vi "07_dosing.vi"() -> ()   [LabVIEW 2024]
uses:
  <vilib>/Utility/error.llb/DialogType.ctl
  4067e6f5-c9bb-441e-8d38-abed3cce061a.vi
  <vilib>/Waveform/WDTOps.llb/WDT Get XY Value DBL.vi
  <vilib>/Utility/file.llb/Write Delimited Spreadsheet (DBL).vi
  <instrlib>/Tektronix DMM40x0 Series/Tektronix DMM40x0 Series.lvlib
panel:
  in  "stop":bool
  out "STABLE":bool
  in  "Serial Communication":T1={"Baud Rate"=9600, "Parity"=0, "Data Bits"=8, "Stop Bits"=10, "Flow Control"=0} {"Flow Control" items=["None", "XON/XOFF", "RTS/CTS", "XON/XOFF & RTS/CTS", "DTR/DSR", "XON/XOFF & DTR/DSR"]; "Stop Bits" items=["1.0"=10, "1.5"=15, "2.0"=20]; "Data Bits" items=["7"=7, "8"=8]; "Parity" items=["None", "Odd", "Even", "Mark", "Space"]; "Baud Rate" items=["300"=300, "600"=600, "1200"=1200, "2400"=2400, "4800"=4800, "9600"=9600, "19200"=19200]}
  out "Stability threshold":dbl format="%#_13g"
  out "Waveform Graph":dbl[](graph)
  # "Voltmeter Serial Configuration"
  # "DEFAULT SETTINGS:\n\nTimeout (10000 ms)\nTrigger Count (5000)\nSample Count (1)\n\n****DC VOLTAGE***"
  # "Voltmeter Stability"
  # "0 - Stability threshold not met\n1 - Stability threshold met\n\n\n\n*stability (+/-0.05 mV) of last 15 pts"
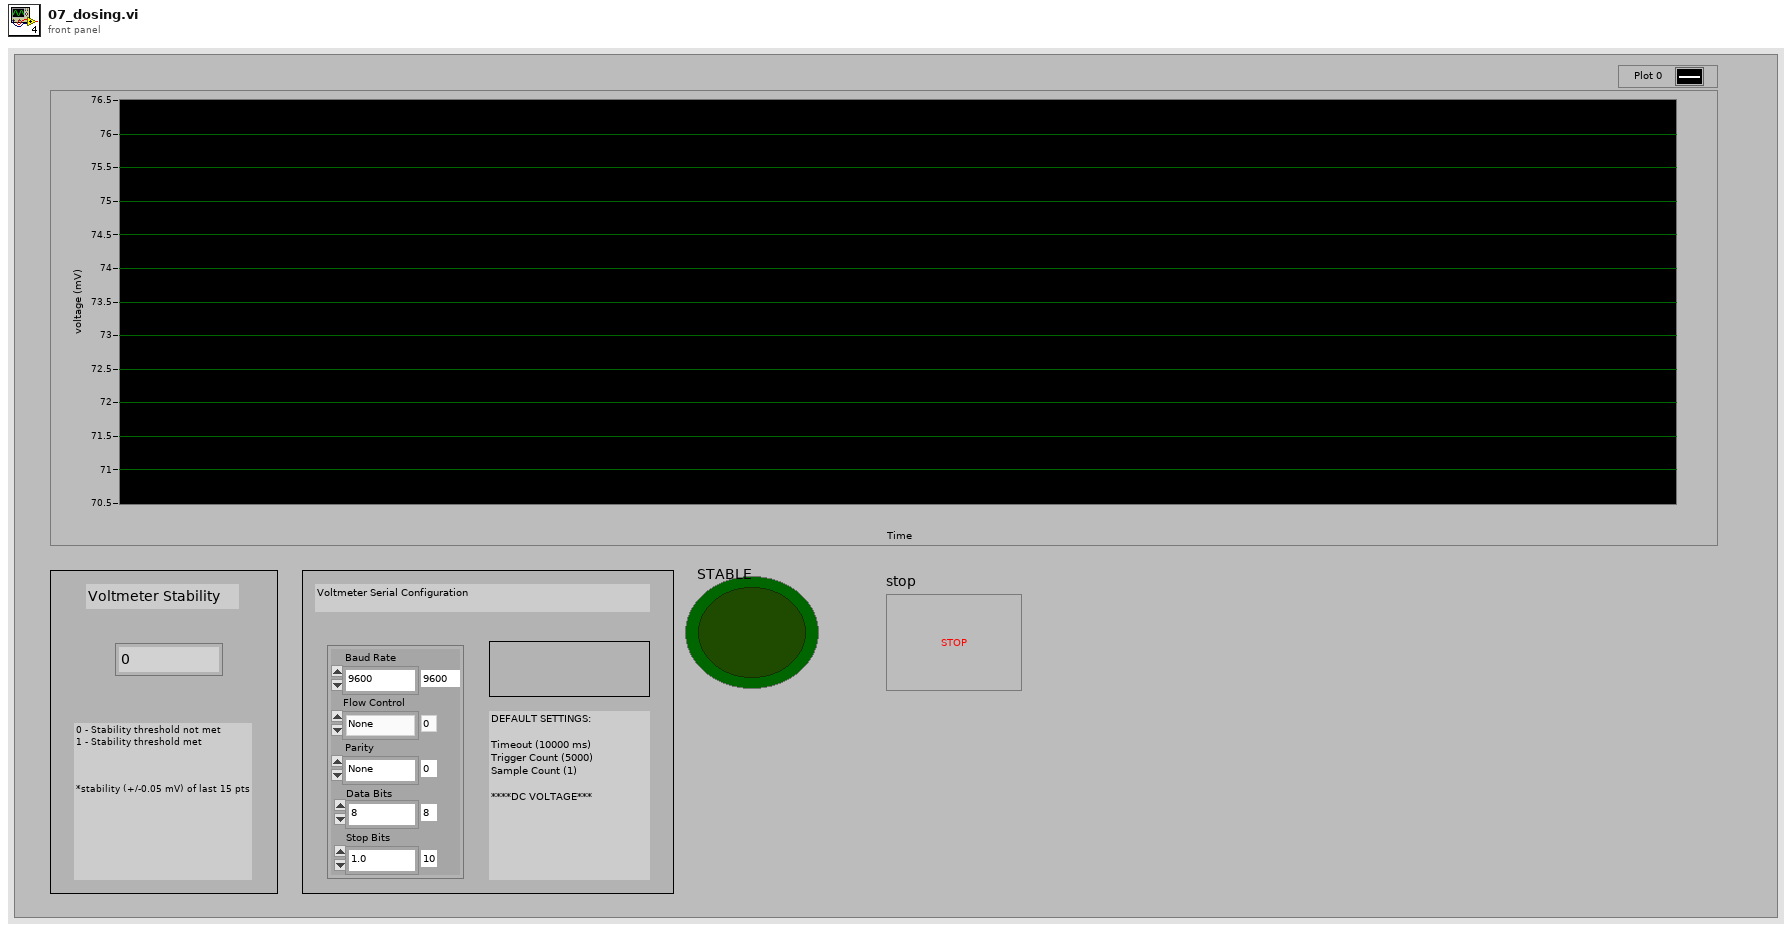
[diagram p1: front panel]
types:
  T1 = cluster{"Baud Rate":u32, "Parity":u16, "Data Bits":u16, "Stop Bits":u16, "Flow Control":u16}
  T2 = typedef "DialogType.ctl" = u16
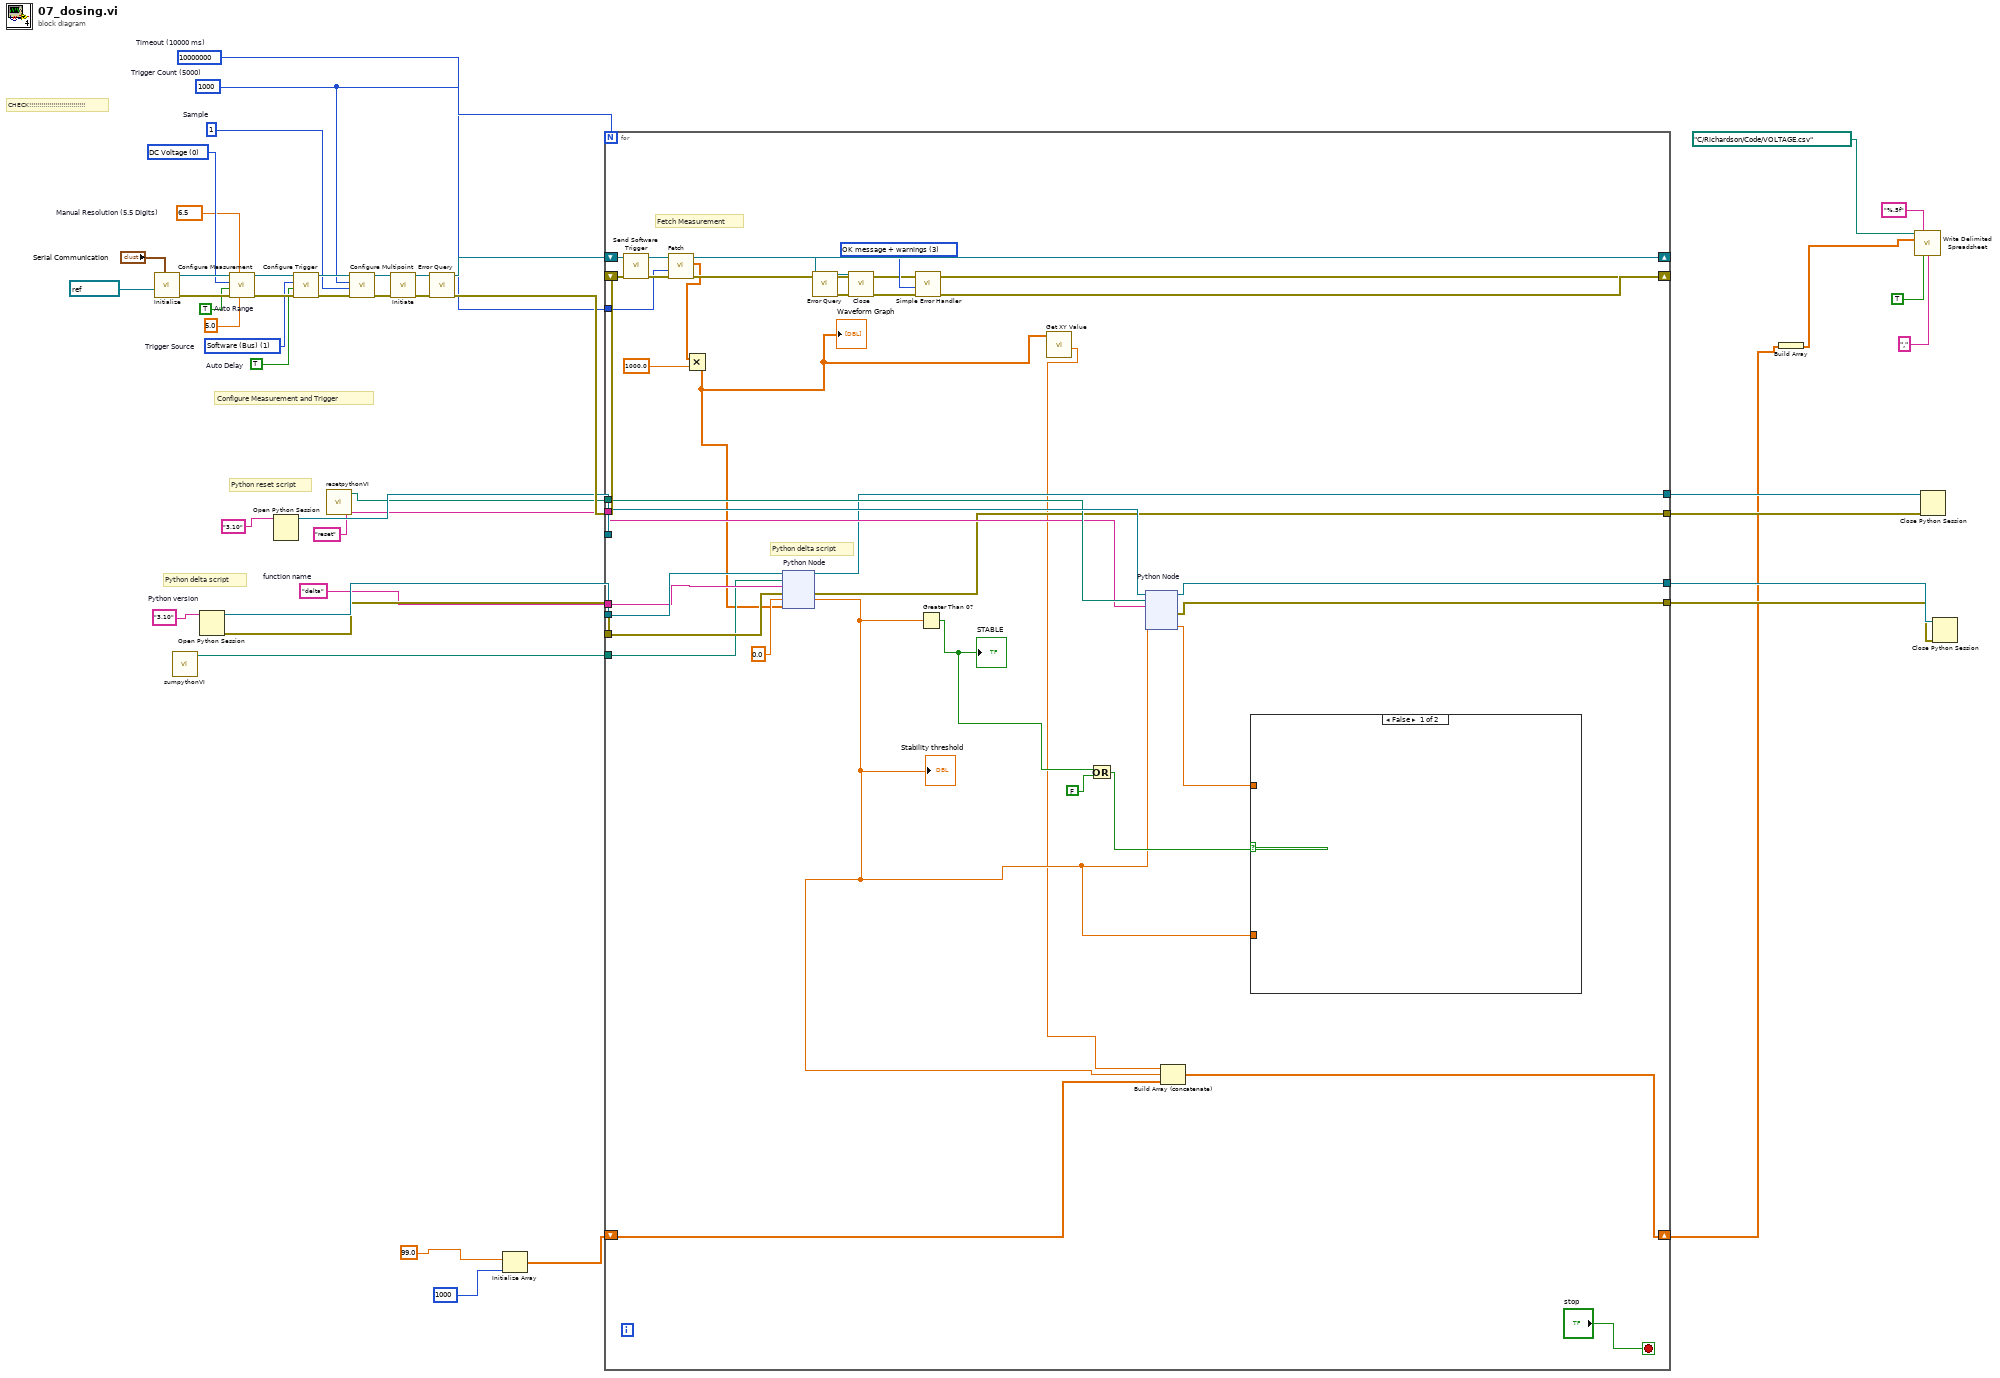
[diagram p0: block diagram]
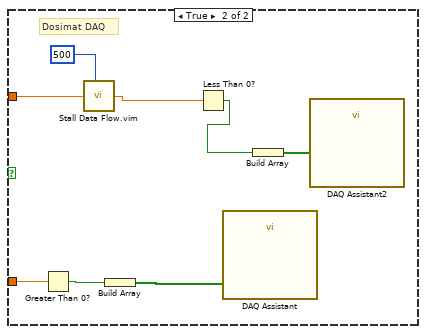
[diagram p2: hidden frame]
diagram:
  w10 = T2 3 items=["no dialog", "OK message", "continue or stop message", "OK message + warnings", "continue/stop + warnings"] ("type of dialog (OK msg:1)")
  w23 = "delta"  # function name
  w26 = "3.10"  # Python version
  w38 = u16 0 items=["DC Voltage", "AC Voltage", "2 - Wire Resistance", "4 - Wire Resistance", "DC Current", "AC Current", "Frequency", "Period", "Continuity", "Diode Checking", "Temperature", "Capacitance"] ("Function (0: DC Voltage)")
  w29 = u32 10000000  # Timeout (10000 ms)
  w30 = 1  # Sample
  w37 = 1000  # Trigger Count (5000)
  w31 = 6.5 items=["4.5"=4.5, "5.5"=5.5, "6.5"=6.5]  # Manual Resolution (5.5 Digits)
  w39 = TRUE  # Auto Delay
  w40 = u16 1 items=["Immediate", "Software (Bus)", "External"]  # Trigger Source
  w41 = TRUE  # Auto Range
  # "Python delta script"
  # "Python reset script"
  # "CHECK!!!!!!!!!!!!!!!!!!!!!!!!!!!!"
  # "Configure Measurement and Trigger"
  n1 = call <instrlib>:"Initialize.vi"("Serial Configuration"="Serial Communication", "VISA resource name"=refnum<visa-resource-name> "COM2" ("COM PORT (COM2)")) -> ("error out"=w50:errorcluster, "VISA resource name out"=w51:refnum<visa-resource-name>)  [unwired: 3 in, 5 out]
  n2 = call "sumpythonVI.vi"() -> ("appended path"=w22:path)  [unwired: 11 in]
  n3 = Open Python Session(python version=w26) -> (session out=w28:refnum<k35>, error out=w27:errorcluster)  [unwired: 2 in]
  n4 = call <instrlib>:"Configure Measurement.vi"("Manual Range (1.0)"=5.0, "Manual Resolution (5.5 Digits)"=w31, "error in (no error)"=w50, "Auto Range (T:Enable)"=w41, "Function (0: DC Voltage)"=w38, "VISA resource name"=w51) -> ("error out"=w48:errorcluster, "VISA resource name out"=w49:refnum<visa-resource-name>)  [unwired: 4 out]
  n5 = Open Python Session(python version="3.10" ("Python version")) -> (session out=w24:refnum<k35>)  [unwired: 2 in, 1 out]
  n6 = call <instrlib>:"Configure Trigger.vi"("error in (no error)"=w48, "Auto Delay (T: Enable)"=w39, "Trigger Source (0: Immediate)"=w40, "VISA resource name"=w49) -> ("error out"=w46:errorcluster, "VISA resource name out"=w47:refnum<visa-resource-name>)  [unwired: 1 in, 5 out]
  n7 = call "resetpythonVI.vi"() -> ("appended path"=w21:path)  [unwired: 11 in]
  n8 = call <instrlib>:"Configure Multipoint.vi"("error in (no error)"=w46, "Sample Count (1)"=w30, "Trigger Count (1)"=w37, "VISA resource name"=w47) -> ("error out"=w44:errorcluster, "VISA resource name out"=w45:refnum<visa-resource-name>)  [unwired: 6 out]
  n9 = call <instrlib>:"Initiate.vi"("error in (no error)"=w44, "VISA resource name"=w45) -> ("error out"=w36:errorcluster, "VISA resource name out"=w35:refnum<visa-resource-name>)  [unwired: 8 out]
  n10 = call <instrlib>:"Error Query.vi"("error in (no error)"=w36, "VISA resource name"=w35) -> ("error out"=w33:errorcluster, "VISA resource name out"=w34:refnum<visa-resource-name>)  [unwired: 8 out]
  n11 = Initialize Array(99.0 ("element"), 1000 ("dimension size")) -> (w4:dbl[])
  n12 = for {
    N: w37 -> [_]
    shift-right: [w81] -> w12
    shift-left: w33 -> [w77]
    shift-right: [w82] -> w14
    shift-left: w34 -> [w78]
    tunnel: w29 -> [w76]
    tunnel: w28 -> [w71]
    tunnel: w27 -> [w70]
    tunnel: w24 -> [w69]
    tunnel: w23 -> [w68]
    tunnel: w22 -> [w67]
    tunnel: w21 -> [w66]
    tunnel: "reset" ("function name") -> [w65]
    tunnel: [w64] -> w19
    tunnel: [w63] -> w18
    tunnel: [w62] -> w17
    tunnel: [w61] -> w16
    shift-right: [w57] -> w2
    shift-left: w4 -> [w54]
    stop <- "stop" stop-if-true
    # "Python delta script"
    # "Fetch Measurement"
    n13 = call <instrlib>:"Send Software Trigger.vi"("error in (no error)"=w77, "VISA resource name"=w78) -> ("error out"=w79:errorcluster, "VISA resource name out"=w80:refnum<visa-resource-name>)  [unwired: 8 out]
    n14 = call <instrlib>:"Fetch.vi"("error in (no error)"=w79, "Timeout (10000 ms)"=w76, "VISA resource name"=w80) -> ("error out"=w81:errorcluster, "Measurements"=w74:dbl[], "VISA resource name out"=w82:refnum<visa-resource-name>)  [unwired: 6 out]
    n15 = Multiply(x=w74, y=1000.0) -> (x*y=w53:dbl[])
    "Waveform Graph" <- w53
    n16 = node "Python Node"(w71, w67, w68, w70, 0.0, w53) -> (w62:refnum<k35>, w61:errorcluster, w55:dbl)  [unwired: 1 in, 2 out]
    "Stability threshold" <- w55
    n17 = Greater Than 0?(x=w55) -> (x > 0?=w58:bool)
    "STABLE" <- w58
    n18 = call-poly <vilib>:"Get XY Value.vi"("waveform in"=w53) -> ("Y value"=w52:dbl)  [unwired: 6 in, 4 out]
    n19 = Or(x=w58, y=FALSE) -> (x .or. y?=w56:bool)
    n20 = node "Python Node"(w69, w66, w65, w55) -> (w64:refnum<k35>, w63:errorcluster, w72:dbl)  [unwired: 3 in, 2 out]
    n21 = Build Array (concatenate)(w52, w55, w54) -> (w57:dbl[])
    n22 = case shown="False" w56 {
      tunnel: w72 -> [_ w85]
      tunnel: w55 -> [_ w83]
      frame False {
      }
      frame True {
        # "Dosimat DAQ"
        n23 = Greater Than 0?(x=w83) -> (x > 0?=w88:bool)
        n24 = call "Stall Data Flow.vim"("value in"=w85, "milliseconds to wait"=u32 500) -> ("value out"=w86:dbl)  [unwired: 1 out]
        n25 = Build Array(w88) -> (w87:bool[])
        n26 = Less Than 0?(x=w86) -> (x < 0?=w89:bool)
        n27 = call "DAQ Assistant"("data"=w87) -> ()  [unwired: 17 in, 2 out]
        n28 = Build Array(w89) -> (w90:bool[])
        n29 = call "DAQ Assistant2"("data"=w90) -> ()  [unwired: 17 in, 2 out]
      }
    }
  }
  n30 = call <instrlib>:"Error Query.vi"("error in (no error)"=w12, "VISA resource name"=w14) -> ("error out"=w11:errorcluster, "VISA resource name out"=w13:refnum<visa-resource-name>)  [unwired: 8 out]
  n31 = call <instrlib>:"Close.vi"("error in (no error)"=w11, "VISA resource name"=w13) -> ("error out"=w15:errorcluster)  [unwired: 9 out]
  n32 = call <vilib>:"Simple Error Handler.vi"("type of dialog (OK msg:1)"=w10, "error in (no error)"=w15) -> ()  [unwired: 8 out]
  n33 = Build Array(w2) -> (w3:dbl[][])
  n34 = call-poly <vilib>:"Write Delimited Spreadsheet.vi"("file path (dialog if empty)"=path "C:/Richardson/Code/VOLTAGE.csv", "format (%.3f)"="%.5f", "2D data"=w3, "transpose? (no:F)"=TRUE, "delimiter (\\t)"="," ("delimiter (\\t)")) -> ()  [unwired: 9 in, 2 out]
  n35 = Close Python Session(session in=w17, error in=w16) -> ()  [unwired: 1 out]
  n36 = Close Python Session(session in=w19, error in=w18) -> ()  [unwired: 1 out]
